vi "instance count allowed.vi"(8 "error in":errorcluster, 11 "asynchronous execution component configuration in":refnum<class "asynchronous execution module configuration.lvclass">) -> (0 "error out":errorcluster, 2 "instances allowed":i32, 3 "asynchronous execution component configuration out":refnum<class "asynchronous execution module configuration.lvclass">)   [LabVIEW 2013, in "asynchronous execution module configuration.lvclass"]
doc: "An accessor method which indicates the number of instances of a runtime class which should be allowed to execute in a given application instance or system. The component has no use for this information--it may only be acted upon by calling code."
uses:
  asynchronous execution module configuration.lvclass
  asynchronous execution module configuration.lvclass/asynchronous execution module configuration.ctl
  <vilib>/NI/Tag Bus Module Framework/module configuration/TBM module configuration.lvclass
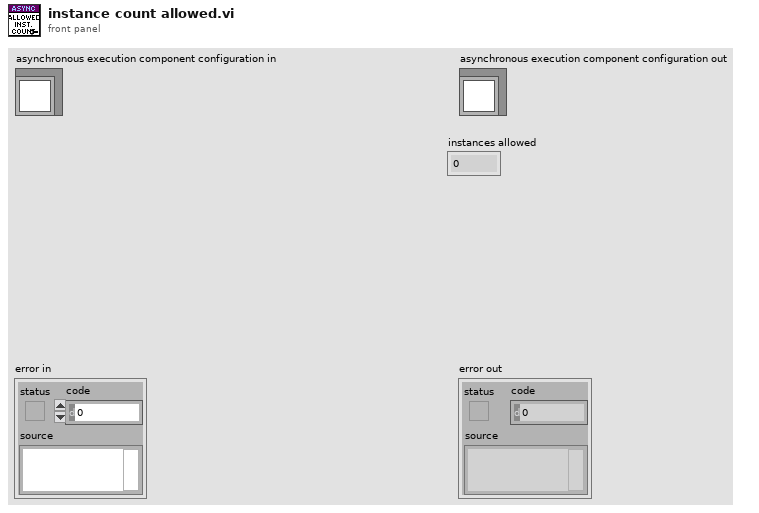
[diagram p1: front panel]
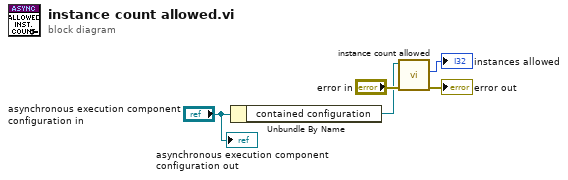
[diagram p0: block diagram]
diagram:
  n1 = Unbundle By Name("asynchronous execution component configuration in") -> ("contained configuration"=w1:refnum<class "TBM module configuration.lvclass">)
  n2 = call-dynamic "instance count allowed.vi"("error in"="error in", "module configuration in"=w1) -> ("error out"=→"error out":errorcluster, "instances allowed"=→"instances allowed":i32)  [unwired: 7 in, 1 out]
  "asynchronous execution component configuration out" <- "asynchronous execution component configuration in"
